vi "Read Device.lvclass.vi"(11 "Measurements in":refnum<class "Measurement.lvclass">) -> (2 "Device.lvclass":refnum<class "Device.lvclass">, 3 "Measurements out":refnum<class "Measurement.lvclass">)   [LabVIEW 2020, in "Measurement.lvclass"]
uses:
  Measurement.lvclass
  Devices/Device.lvclass
  Measurement.lvclass/Measurement.ctl
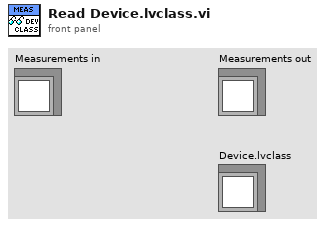
[diagram p1: front panel]
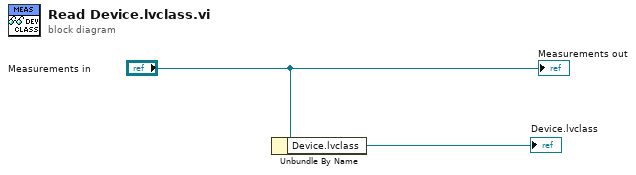
[diagram p0: block diagram]
diagram:
  n1 = Unbundle By Name("Measurements in") -> ("Device.lvclass"=→"Device.lvclass":refnum<class "Device.lvclass">)
  "Measurements out" <- "Measurements in"
